vi "Peak Detection and Display.vi"() -> ()   [LabVIEW 2020]
doc: "Demonstrates the use of the Peak Detector VI."
uses:
  <vilib>/Analysis/NI_AALBase.lvlib
  <vilib>/Analysis/NI_AAL_SigProc.lvlib
  <vilib>/Analysis/3filter.llb/Elliptic Filter (DBL).vi
panel:
  in  "signal source":u16(ring) items=["Filtered Noise", "Sinc", "Sin + Cos"]
  out "valleys found":i32
  in  "Stop":bool
  in  "filter order":i32=2
  in  "noise seed":i32=1
  in  "peak detector width":i32=3 min=3
  out "Signal Plot":cluster{"Locations":dbl[], "Amplitudes":dbl[]}[](graph)
  out "peaks found":i32
  # "Overview: Demonstrates the use of the Peak Detector VI to find peaks and valleys in a variety of signals.\nRequirements: LabVIEW Full Development System\nInstructions:\n1. Run the VI.\n2. Within the Signal Plot, move the horizontal cursors to adjust the peak detector threshold levels (red for Peaks, blue for Valleys).\n3. Change the signal source along with the noise seed and filter order to modify the signal shape.\n4. Change the peak detector width to observe how smoothing increases with width.\n5. Click Stop to stop the VI."
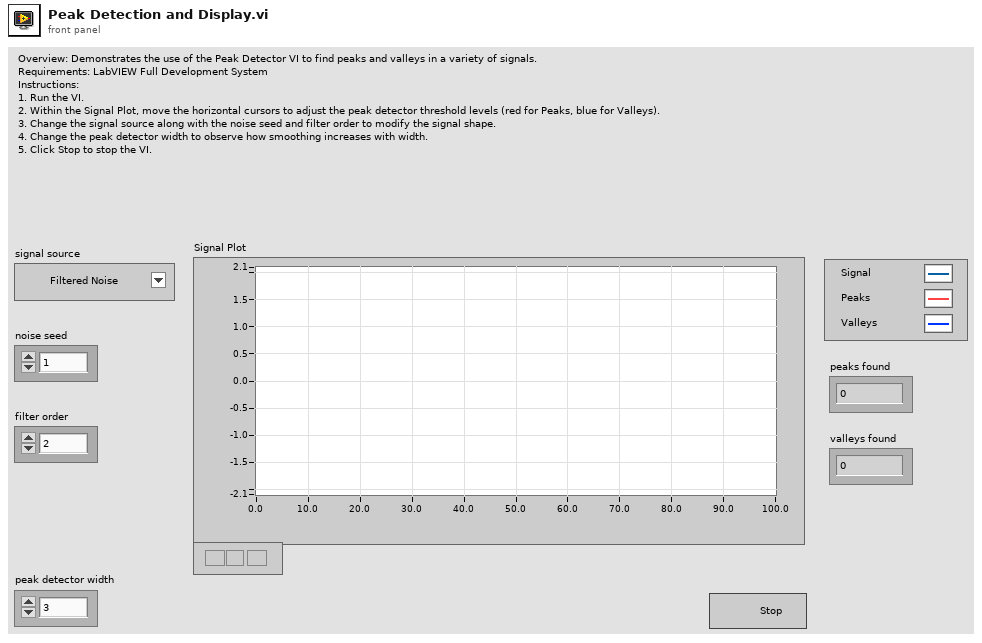
[diagram p1: front panel]
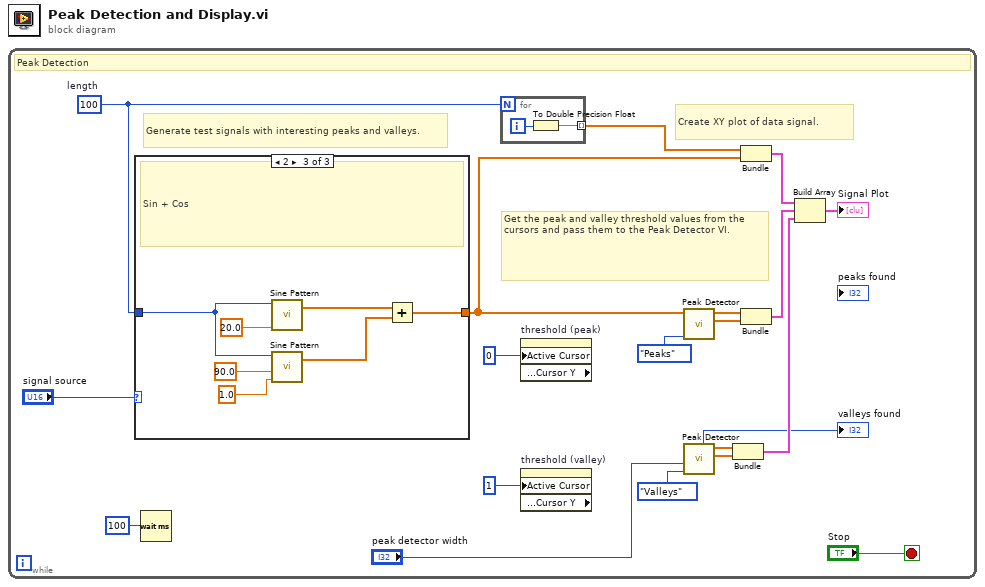
[diagram p0: block diagram]
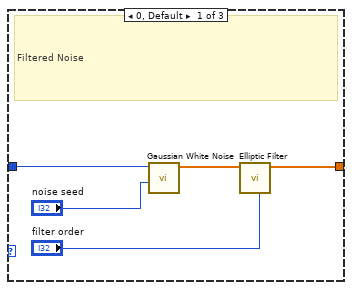
[diagram p2: hidden frame]
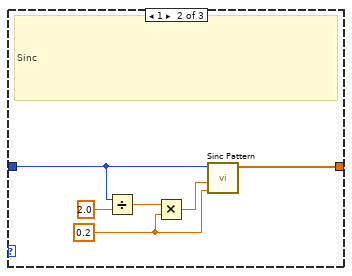
[diagram p3: hidden frame]
diagram:
  n1 = while {
    stop <- "Stop" stop-if-true
    w7 = 100  # length
    # "Get the peak and valley threshold values from the cursors and pass them to the Peak Detector VI."
    # "Create XY plot of data signal."
    # "Generate test signals with interesting peaks and valleys."
    # "Peak Detection"
    n2 = case shown="2" "signal source" {
      tunnel: [w25 w31 w39] -> w6
      tunnel: w7 -> [w27 w30 w37]
      frame 0, Default {
        # "Filtered Noise"
        n3 = call <vilib>:"Gaussian White Noise.vi"("seed"="noise seed", "samples"=w27) -> ("Gaussian noise pattern"=w26:dbl[])  [unwired: 8 in, 1 out]
        n4 = call-poly <vilib>:"Elliptic Filter.vi"("order"="filter order", "X"=w26) -> ("Filtered X"=w25:dbl[])  [unwired: 8 in, 1 out]
      }
      frame 1 {
        w28 = 0.2
        # "Sinc"
        n5 = Divide(x=w30, y=2.0) -> (x/y=w33:dbl)
        n6 = Multiply(x=w33, y=w28) -> (x*y=w32:dbl)
        n7 = call <vilib>:"Sinc Pattern.vi"("delta t"=w28, "delay"=w32, "samples"=w30) -> ("Sinc Pattern"=w31:dbl[])  [unwired: 1 in, 1 out]
      }
      frame 2 {
        # "Sin + Cos"
        n8 = call <vilib>:"Sine Pattern.vi"("cycles"=20.0, "samples"=w37) -> ("Sinusoidal Pattern"=w40:dbl[])  [unwired: 2 in, 1 out]
        n9 = call <vilib>:"Sine Pattern.vi"("cycles"=1.0, "phase(degrees)"=90.0, "samples"=w37) -> ("Sinusoidal Pattern"=w38:dbl[])  [unwired: 1 in, 1 out]
        n10 = Add(x=w40, y=w38) -> (x+y=w39:dbl[])
      }
    }
    n11 = Wait (ms)(milliseconds to wait=u32 100) -> ()  [unwired: 1 out]
    n12 = for {
      N: w7 -> [_]
      tunnel: [w21] -> w8 mode=indexing
      i -> [w22]
      n13 = To Double Precision Float(number=w22) -> (double precision float=w21:dbl)
    }
    n14 = property on="threshold (peak)" class="XYGraph (strict)" props=["Active Cursor", "Cursor", "Cursor Position:Cursor Y"]("Active Cursor"=u32 0) -> ()  [unwired: 2 in, 3 out]
    n15 = property on="threshold (valley)" class="XYGraph (strict)" props=["Active Cursor", "Cursor", "Cursor Position:Cursor Y"]("Active Cursor"=u32 1) -> ()  [unwired: 2 in, 3 out]
    n16 = call <vilib>:"Peak Detector.vi"("peaks/valleys"=enum32{"Peaks", "Valleys"}."Peaks", "X"=w6) -> ("Amplitudes"=w18:dbl[], "Locations"=w10:dbl[])  [unwired: 5 in, 3 out]
    n17 = call <vilib>:"Peak Detector.vi"("peaks/valleys"=enum32{"Peaks", "Valleys"}."Valleys", "width"="peak detector width") -> ("Amplitudes"=w15:dbl[], "Locations"=w16:dbl[], "# found"=→"valleys found":i32)  [unwired: 5 in, 2 out]
    n18 = Bundle("Locations"=w16, "Amplitudes"=w15) -> (w13:cluster{"Locations":dbl[], "Amplitudes":dbl[]})  [unwired: 1 in]
    n19 = Bundle(w8, "Sinc Pattern"=w6) -> (w20:cluster{dbl[], "Sinc Pattern":dbl[]})  [unwired: 1 in]
    n20 = Bundle("Locations"=w10, "Amplitudes"=w18) -> (w17:cluster{"Locations":dbl[], "Amplitudes":dbl[]})  [unwired: 1 in]
    n21 = Build Array(w20, w17, w13) -> (→"Signal Plot":cluster{"Locations":dbl[], "Amplitudes":dbl[]}[])
  }
